vi "Day 1.1 - Calibration value.vi"(11 "input":string[](array[string])) -> (3 "ouptut part 1":u64)   [LabVIEW 2021]
uses:
  <vilib>/regexp/Match Regular Expression.xnode
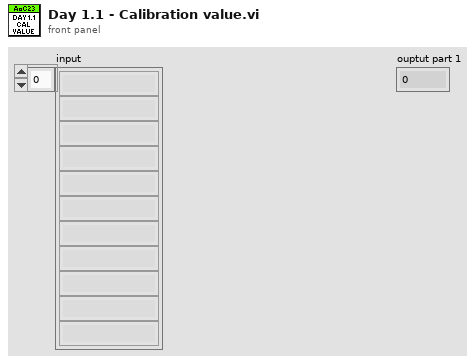
[diagram p1: front panel]
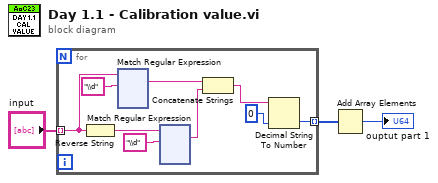
[diagram p0: block diagram]
diagram:
  n1 = for {
    tunnel: "input" -> [w11] mode=indexing
    tunnel: [w5] -> w2 mode=indexing
    n2 = Reverse String(1:w11) -> (0:w9:string)
    n3 = xnode "Match Regular Expression"("input string"=w11, "regular expression"="\\d") -> ("whole match"=w8:string)  [unwired: 4 in, 4 out]
    n4 = xnode "Match Regular Expression"("input string"=w9, "regular expression"="\\d") -> ("whole match"=w7:string)  [unwired: 4 in, 4 out]
    n5 = Concatenate Strings(w8, w7) -> (w6:string)
    n6 = Decimal String To Number(string=w6, default (0L)=u64 0 ("default (0 I32)")) -> (number=w5:u64)  [unwired: 1 in, 1 out]
  }
  n7 = Add Array Elements(numeric array=w2) -> (sum=→"ouptut part 1":u64)
